vi "Dialog.vi"   [LabVIEW 2020, in "2. Basic Panel Actors.lvlib" / "Sample Panel.lvclass"]
doc: "Simple Dialog for testing.\n----\nCopyright: MGI 2017\nAuthor: Derek Trepanier"
uses:
  Sample Panel.lvclass
  <vilib>/MGI/Panel Manager/Panel/Panel/Window/Dialog/Dialog.lvclass
  C:/Program Files/National Instruments/LabVIEW 2020/vi.lib/MGI/Panel Manager/Panel/Panel/Panel.lvclass
  <vilib>/MGI/Panel Manager/Panel/Panel.lvlib
  <vilib>/MGI/Panel Manager/Panel/Panel/Panel.lvclass
panel:
  # "Test Dialog"
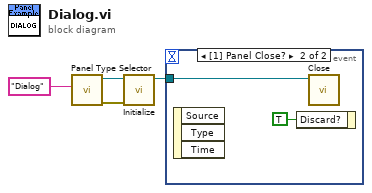
[diagram p0: block diagram]
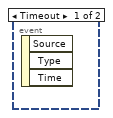
[diagram p2: hidden frame]
diagram:
  n1 = call-poly <vilib>:"Panel Type Selector.vi"("Default Title"="Dialog" ("Title")) -> ("Error Out"=w3:errorcluster, "Dialog out"=w4:refnum<class "Dialog.lvclass">)  [unwired: 9 in]
  n2 = call <vilib>:"Initialize.vi"("error in (no error)"=w3, "Panel In"=w4) -> ("Panel Out"=w1:refnum<class "Dialog.lvclass">)  [unwired: 7 in, 2 out]
  n3 = event shown="[1] Panel Close?" {
    selector: _ -> [_ _]
    dyn-events: _ -> [_ _]
    timeout: _ -> [_ _]
    tunnel: w1 -> [_ w6]
    event Timeout {
      n4 = event-data() -> ()  [unwired: 1 in, 3 out]
    }
    event Panel Close? {
      n5 = event-data() -> ()  [unwired: 1 in, 3 out]
      n6 = event-data("Discard?"=TRUE) -> ()  [unwired: 1 in, 1 out]
      n7 = call-dynamic "Close.vi"("Dialog in"=w6) -> ()  [unwired: 10 in, 1 out]
    }
  }
